vi "Build Call Chain.vi"() -> (1 "Call Chain":string)   [LabVIEW 2020, in "WebServiceImporter.lvlib" / "Error Handling.lvlib"]
uses:
  <vilib>/Platform/WebService/Error Handling/Error Handling.lvlib
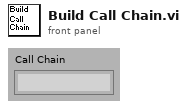
[diagram p1: front panel]
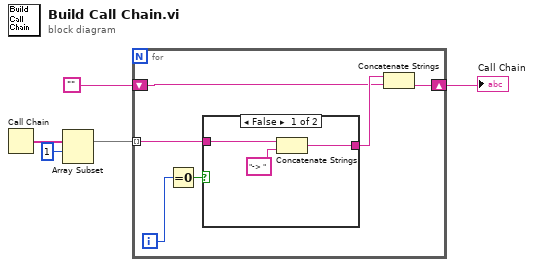
[diagram p0: block diagram]
diagram:
  n1 = Call Chain() -> (call chain=w5:string[])
  n2 = Array Subset(array=w5, index=1) -> (w3:string[])  [unwired: 1 in]
  n3 = for {
    tunnel: w3 -> [w9] mode=indexing
    shift-right: [w8] -> w1
    shift-left: "" -> [w6]
    i -> [w11]
    n4 = Equal To 0?(x=w11) -> (x = 0?=w10:bool)
    n5 = case shown="False" w10 {
      tunnel: w9 -> [w13 w15]
      tunnel: [w14 w15] -> w7
      frame False {
        n6 = Concatenate Strings(w13, "-> " ("string")) -> (w14:string)
      }
      frame True {
      }
    }
    n7 = Concatenate Strings(w7, w6) -> (w8:string)
  }
  "Call Chain" <- w1
